vi "AssertsSubpanelVIExec.vi"(0 "VI Reference In":refnum<vi>, 1 "Label (VI Title)":string="Default", 11 "error in":errorcluster) -> (4 "VI Reference Out":refnum<vi>, 15 "error out":errorcluster)   [LabVIEW 2016, in "DronaTest.lvlib"]
uses:
  DronaTest.lvlib
  APIs/Assert/AssertSubpanel/AssertSubpanelVIExecRunning.vi
  APIs/Stimulus/ControlValue/ValueSignalLatchBooleanString.vi
  APIs/Assert/AssertSubpanel/AssertSubpanelVIExecIdle.vi
  <vilib>/addons/_JKI Toolkits/Caraya/classes/Assert/Assert Not Error.vi
  <vilib>/addons/_JKI Toolkits/Caraya/classes/Test/Test.lvclass
  Drona.lvlib
  <vilib>/addons/_JKI Toolkits/Caraya/classes/Assert/Assert.lvclass
  APIs/Assert/AssertSubpanel/AssertSubpanel.lvlib
  APIs/Stimulus/ControlValue/ControlValue.lvlib
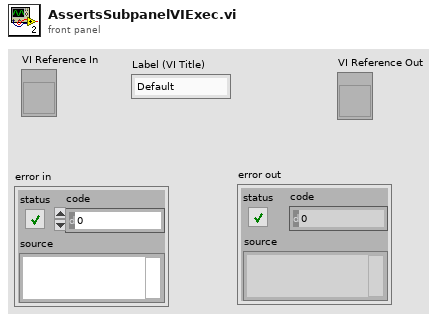
[diagram p1: front panel]
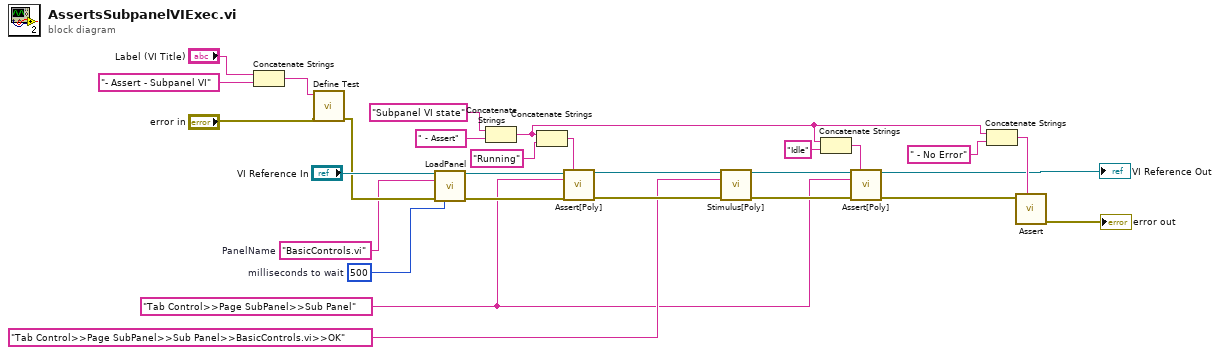
[diagram p0: block diagram]
diagram:
  w18 = u32 500  # milliseconds to wait
  w19 = "BasicControls.vi"  # PanelName
  w6 = "Tab Control>>Page SubPanel>>Sub Panel" ("Control Path")
  n1 = Concatenate Strings("Label (VI Title)", "- Assert - Subpanel VI" ("string")) -> (w25:string)
  n2 = call <vilib>:"Define Test.vi"("error in (no error)"="error in", "Label (VI Title)"=w25) -> ("error out"=w20:errorcluster)  [unwired: 9 in]
  n3 = call "LoadPanel.vi"("VI in"="VI Reference In", "Panel Name"=w19, "error in (no error)"=w20, "milliseconds to wait"=w18) -> ("VI out"=w15:refnum<vi>, "error out"=w14:errorcluster)  [unwired: 10 in]
  n4 = Concatenate Strings("Subpanel VI state" ("Label"), " - Assert" ("string")) -> (w1:string)
  n5 = Concatenate Strings(w1, "Running" ("string")) -> (w4:string)
  n6 = call-poly "Assert[Poly].vi"("VI Reference In"=w15, "Test Label"=w4, "Control Path"=w6, "Error In"=w14) -> ("VI Reference Out"=w12:refnum<vi>, "Error Out"=w13:errorcluster)  [unwired: 10 in]
  n7 = call-poly "Stimulus[Poly].vi"("VI Reference In"=w12, "Control Path"="Tab Control>>Page SubPanel>>Sub Panel>>BasicControls.vi>>OK", "error in"=w13) -> ("VI Reference Out"=w10:refnum<vi>, "error out"=w8:errorcluster)  [unwired: 11 in]
  n8 = Concatenate Strings(w1, "Idle" ("string")) -> (w3:string)
  n9 = call-poly "Assert[Poly].vi"("VI Reference In"=w10, "Test Label"=w3, "Control Path"=w6, "Error In"=w8) -> ("VI Reference Out"=→"VI Reference Out":refnum<vi>, "Error Out"=w7:errorcluster)  [unwired: 10 in]
  n10 = Concatenate Strings(w1, " - No Error" ("string")) -> (w28:string)
  n11 = call-poly <vilib>:"Assert.vi"("Label"=w28, "Not Error?"=w7) -> ("error out"=→"error out":errorcluster)  [unwired: 9 in]
